vi "Write.vi"(0 "Message":string, 2 "Que name":string, 5 "error in":errorcluster, 7 "Data":variant, 9 "Priority message?":bool) -> (6 "error out":errorcluster)   [LabVIEW 2014, in "Que lib.lvlib"]
uses:
  Que lib.lvlib
  Controls/Queue cluster.ctl
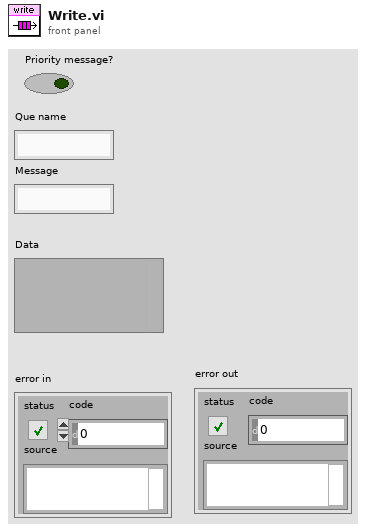
[diagram p1: front panel]
types:
  T1 = typedef "Que lib.lvlib/Queue cluster.ctl" = cluster{"Message":string, "Data":variant}
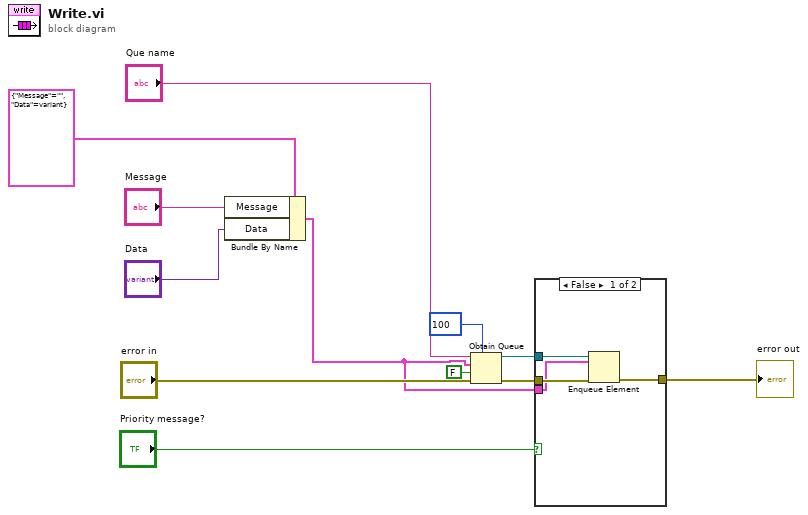
[diagram p0: block diagram]
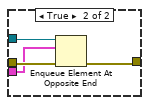
[diagram p2: hidden frame]
diagram:
  n1 = Bundle By Name(cluster=T1 {"Message"="", "Data"=variant} ("Queue Cluster"), "Message"="Message", "Data"="Data") -> (w2:T1)
  n2 = Obtain Queue(max queue size (-1, unlimited)=100, name (unnamed)="Que name", element data type=w2, create if not found? (T)=FALSE, error in (no error)="error in") -> (queue out=w6:refnum<queue>, error out=w12:errorcluster)  [unwired: 1 out]
  n3 = case shown="False" "Priority message?" {
    tunnel: w12 -> [w16 w20]
    tunnel: [w15 w17] -> w10
    tunnel: w6 -> [w14 w19]
    tunnel: w2 -> [w13 w18]
    frame False {
      n4 = Enqueue Element(queue=w14, element=w13, error in (no error)=w16) -> (error out=w15:errorcluster)  [unwired: 1 in, 2 out]
    }
    frame True {
      n5 = Enqueue Element At Opposite End(queue=w19, element=w18, error in (no error)=w20) -> (error out=w17:errorcluster)  [unwired: 1 in, 2 out]
    }
  }
  "error out" <- w10
